vi "Strain Configure Quarter Bridge.vi"(6 "ChannelList":string, 7 "Resolution":dbl, 8 "error in (no error)":errorcluster {"code" format="%.0x"}, 9 "Range":dbl, 10 "GaugeFactor":dbl, 11 "instrument handle":refnum<k15>) -> (0 "error out":errorcluster {"code" format="%.0x"}, 3 "instrument handle out":refnum<k15>)   [LabVIEW 2020, in "Keysight DAQ970.lvlib"]
doc: "Configures the specified channels for quarter bridge strain gauge measurement, but does not initiate a scan. This command redefines the scan list."
uses:
  Keysight DAQ970.lvlib
  KtDAQ970.dll
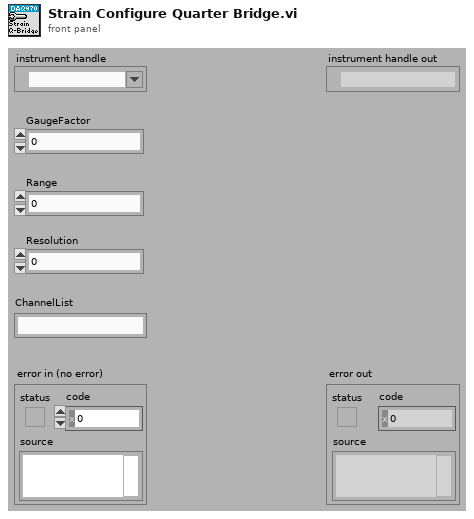
[diagram p1: front panel]
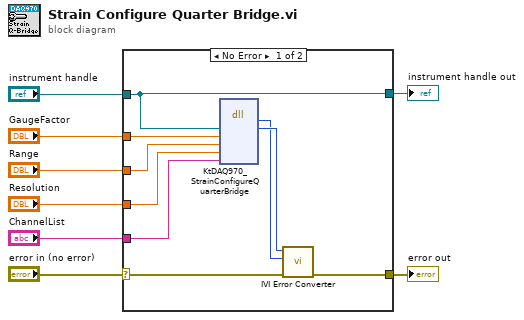
[diagram p0: block diagram]
diagram:
  n1 = case shown="No Error" "error in (no error)" {
    selector: "error in (no error)" -> [w15 w19]
    tunnel: [w14 w19] -> w8
    tunnel: "instrument handle" -> [w9 w18]
    tunnel: "GaugeFactor" -> [w13 _]
    tunnel: "Range" -> [w12 _]
    tunnel: "Resolution" -> [w11 _]
    tunnel: "ChannelList" -> [w10 _]
    tunnel: [w9 w18] -> w1
    frame No Error {
      n2 = dll-call lib="KtDAQ970**.dll" fn="KtDAQ970_StrainConfigureQuarterBridge"("Vi"=w9, "GaugeFactor"=w13, "Range"=w12, "Resolution"=w11, "ChannelList"=w10) -> (w16:i32, "Vi"=w17:u32)  [unwired: 7 in, 2 out]
      n3 = call "IVI Error Converter.vi"("error in (no error)"=w15, "IVI error code (0)"=w16, "instrument handle"=w17) -> ("error out"=w14:errorcluster)  [unwired: 7 in, 1 out]
    }
    frame Error {
    }
  }
  "error out" <- w8
  "instrument handle out" <- w1
